vi "closeFile.vi"(8 "error in (no error)":errorcluster, 11 "Handler.File.Text in":refnum<class "Handler.File.Text.lvclass">) -> (0 "error out":errorcluster, 3 "Handler.File.Text out":refnum<class "Handler.File.Text.lvclass">)   [LabVIEW 2017, in "Error Log.lvlib" / "Handler.File.Text.lvclass"]
uses:
  Handler.File.Text.lvclass
  Handler.File.Text.lvclass/Handler.File.Text.ctl
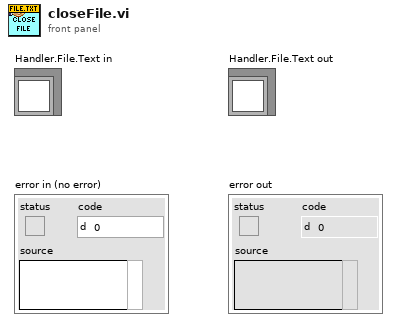
[diagram p1: front panel]
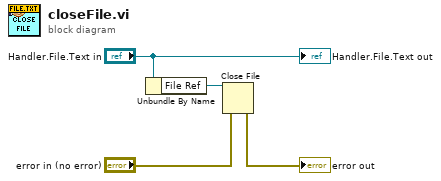
[diagram p0: block diagram]
diagram:
  n1 = Unbundle By Name("Handler.File.Text in") -> ("File Ref"=w3:refnum<file>)
  n2 = Close File(refnum=w3, error in="error in (no error)") -> (error out=→"error out":errorcluster)  [unwired: 1 out]
  "Handler.File.Text out" <- "Handler.File.Text in"
